vi "verify exposure time.vi"(8 "error in (no error)":errorcluster, 11 "Simulated_CCD_Camera in":refnum<class "Sim_Ixon_Ultra.lvclass">) -> (0 "error out":errorcluster, 3 "Simulated_CCD_Camera out":refnum<class "Sim_Ixon_Ultra.lvclass">)   [LabVIEW 2018, in "Sim_Ixon_Ultra.lvclass"]
uses:
  Sim_Ixon_Ultra.lvclass
  C:/Users/Denis/Desktop/S4ACS/S4ACS/Simulated_CCD_Camera/Simulated Camera.lvclass
  Sim_Ixon_Ultra.lvclass/Sim_Ixon_Ultra.ctl
  Simulated_CCD_Camera/Simulated Camera.lvclass
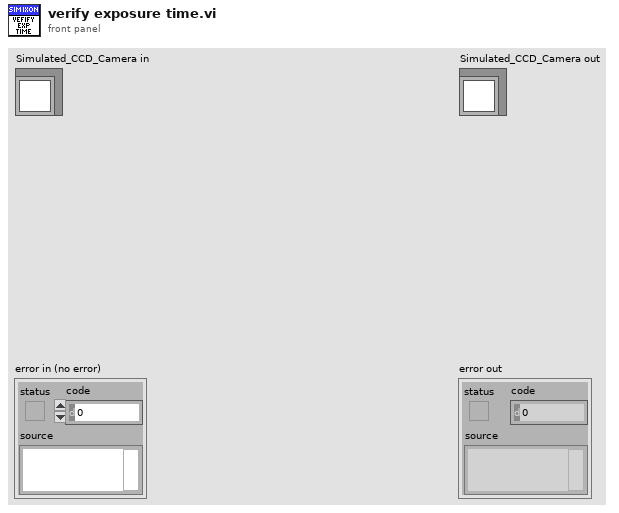
[diagram p1: front panel]
types:
  T1 = typedef "LVDateTimeRec.ctl" = cluster{"fractional second":dbl, "second":i32, "minute":i32, "hour":i32, "day of month":i32, "month":i32, "year":i32, "day of week":i32, "day of year":i32, "DST":i32}
  T2 = cluster{"Time Acq Started":u32, "Image delay":u64, "Last update - CCD config":timestamp, "SYSTEMTIME":T1, "Readout time":dbl, "Time acq finished":u32, "effective exptime":dbl}
  T3 = cluster{"EXPTIME":errorcluster, "#FRAMES":errorcluster}
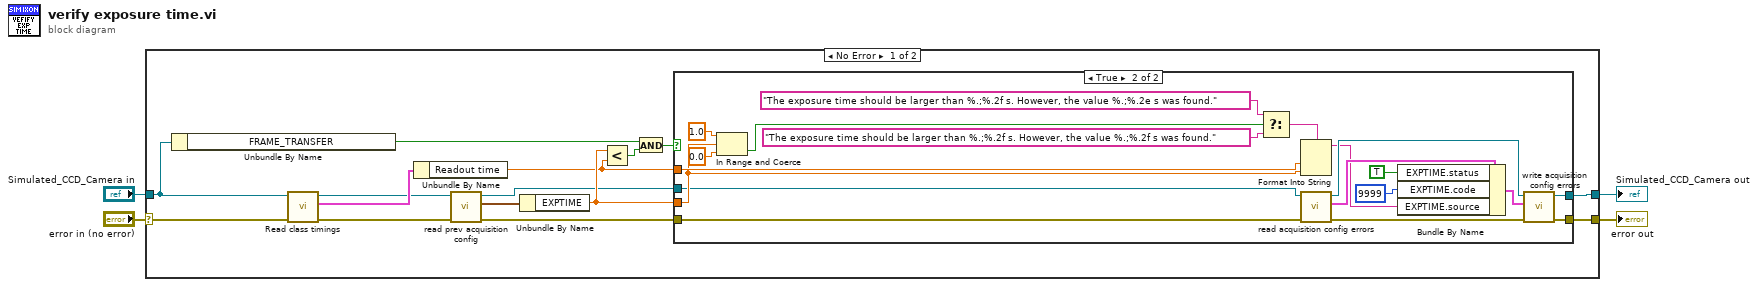
[diagram p0: block diagram]
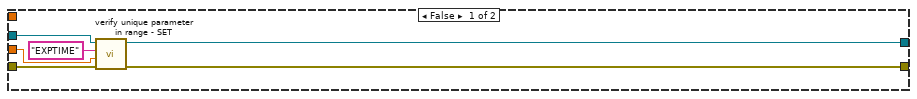
[diagram p2: hidden frame]
diagram:
  n1 = case shown="No Error" "error in (no error)" {
    selector: "error in (no error)" -> [w8 w46]
    tunnel: [w15 w46] -> w3
    tunnel: [w16 w45] -> w2
    tunnel: "Simulated_CCD_Camera in" -> [w11 w45]
    frame No Error {
      n2 = Unbundle By Name(w11) -> ("FRAME_TRANSFER"=w19:bool)
      n3 = call "Read class timings.vi"("error in (no error)"=w8, "Simulated Camera in"=w11) -> ("error out"=w7:errorcluster, "class timings"=w12:T2, "Simulated Camera out"=w10:refnum<class "Sim_Ixon_Ultra.lvclass">)  [unwired: 7 in]
      n4 = Unbundle By Name(w12) -> ("Readout time"=w5:dbl)
      n5 = call "read prev acquisition config.vi"("error in (no error)"=w7, "Simulated_CCD_Camera in"=w10) -> ("error out"=w6:errorcluster, "Prev SET parameters"=w14:cluster{"EXPTIME":dbl, "#FRAMES":u32}, "Simulated_CCD_Camera out"=w9:refnum<class "Sim_Ixon_Ultra.lvclass">)  [unwired: 7 in]
      n6 = Unbundle By Name(w14) -> ("EXPTIME"=w13:dbl)
      n7 = Less?(x=w13, y=w5) -> (x < y?=w18:bool)
      n8 = And(x=w19, y=w18) -> (x .and. y?=w17:bool)
      n9 = case shown="True" w17 {
        tunnel: [w24 w30] -> w16
        tunnel: w6 -> [w22 w33]
        tunnel: w13 -> [w21 w37]
        tunnel: w9 -> [w25 w34]
        tunnel: [w23 w31] -> w15
        tunnel: w5 -> [_ w38]
        frame False {
          n10 = call "verify unique parameter in range - SET.vi"("error in (no error)"=w22, "value"=w21, "parameter name"="EXPTIME", "Simulated_CCD_Camera in"=w25) -> ("error out"=w23:errorcluster, "Simulated_CCD_Camera out"=w24:refnum<class "Sim_Ixon_Ultra.lvclass">)  [unwired: 6 in]
        }
        frame True {
          n11 = In Range and Coerce(upper limit=1.0, x=w37, lower limit=0.0 ("upper limit")) -> (In Range?=w43:bool)  [unwired: 1 out]
          n12 = Select(t="The exposure time should be larger than %.;%.2f s. However, the value %.;%.2e s was found." ("format string"), s=w43, f="The exposure time should be larger than %.;%.2f s. However, the value %.;%.2f s was found." ("format string")) -> (s? t:f=w40:string)
          n13 = Format Into String(format string=w40, w38, w37) -> (resulting string=w29:string)  [unwired: 2 in, 1 out]
          n14 = call "read acquisition config errors.vi"("error in (no error)"=w33, "Simulated Camera in"=w34) -> ("error out"=w26:errorcluster, "acq config errors"=w36:T3, "Simulated Camera out"=w32:refnum<class "Sim_Ixon_Ultra.lvclass">)  [unwired: 7 in]
          n15 = Bundle By Name(cluster=w36, "EXPTIME.status"=TRUE, "EXPTIME.code"=9999 ("SET errors.exposure time.code"), "EXPTIME.source"=w29) -> (w35:T3)
          n16 = call "write acquisition config errors.vi"("error in (no error)"=w26, "SET errors"=w35, "Simulated Camera in"=w32) -> ("error out"=w31:errorcluster, "Simulated Camera out"=w30:refnum<class "Sim_Ixon_Ultra.lvclass">)  [unwired: 7 in]
        }
      }
    }
    frame Error {
    }
  }
  "error out" <- w3
  "Simulated_CCD_Camera out" <- w2
